vi "Curtin1_Color.vi"(8 "Offset":u16, 10 "Files in":T1[](array[typedef]), 11 "Color":u32[](array[colorbox])) -> (2 "New color":u32, 3 "Color palette":u32[](array[colorbox]))   [LabVIEW 2022 SP3]
uses:
  Curtin1_Label.ctl
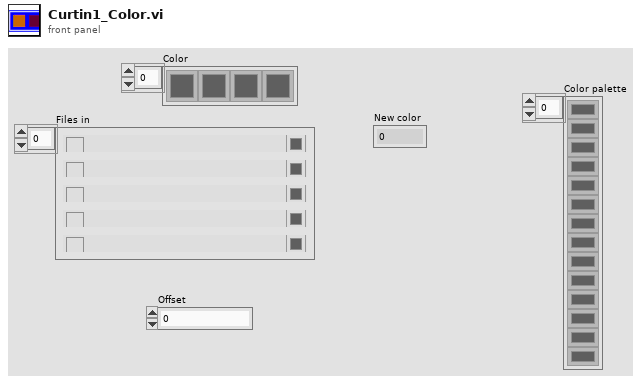
[diagram p1: front panel]
types:
  T1 = typedef "Curtin1_Label.ctl" = cluster{"Show?":bool, "Name":string, "Color":u32, "Path":path, "Show Notes":bool}
  T2 = enum16{"big-endian, network order", "native, host order", "little-endian"}
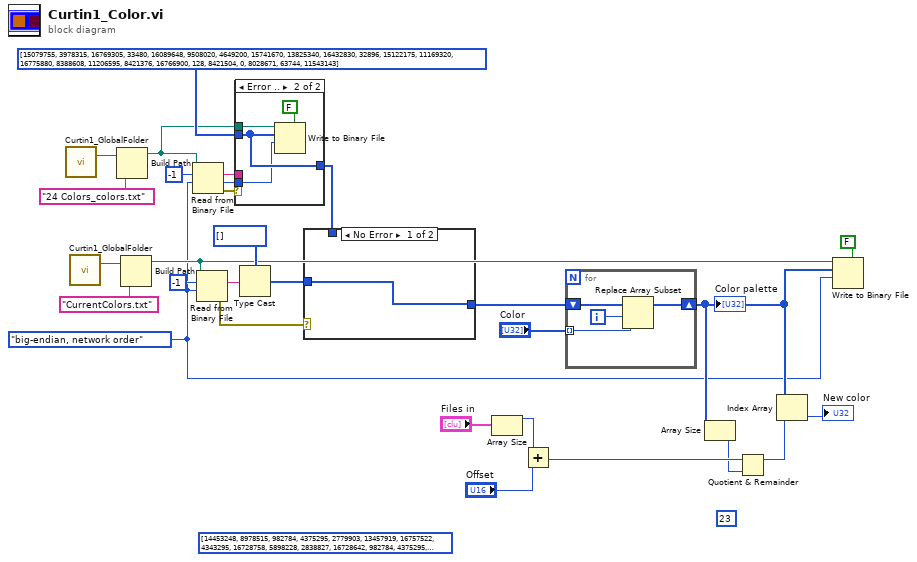
[diagram p0: block diagram]
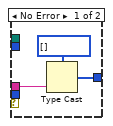
[diagram p2: hidden frame]
diagram:
  w1 = T2."big-endian, network order" ("byte order (0:big-endian, network order)")
  (unwired) 23 ("y")
  (unwired) u32[] [14453248, 8978515, 982784, 4375295, 2779903, 13457919, 16757522, 4343295, 16728758, 5898228, 2838827, 16728642, 982784, 4375295, 13827953, 13457919, 16757522, 4343295, 16728758, 5898228, 16777215, 16728642, 982784, 4375295, 13827953, 13457919, 16757522, 4343295, 16728758, 5898228, 16777215, 16728642, 982784, 4375295, 13827953, 13457919, 16757522, 4343295, 16728758, 5898228, 16777215, 16728642, 982784, 4375295, 13827953, 13457919, 16757522, 4343295, 16728758, 5898228, 16777215, 16728642, 982784, 4375295, 13827953, 13457919, 16757522, 4343295, 16728758, 5898228, 16777215, 16728642, 982784, 4375295, 13827953, 13457919, 16757522, 4343295, 16728758, 5898228, 16777215, 16728642, 982784, 4375295, 13827953, 13457919, 16757522, 4343295, 16728758, 5898228, 16777215, 16728642, 982784, 4375295, 13827953, 13457919, 16757522, 4343295, 16728758, 5898228, 16777215, 16728642, 982784, 4375295, 13827953, 13457919, 16757522, 4343295, 16728758, 5898228] ("Array")
  n1 = call "Curtin1_GlobalFolder.vi"() -> ("LabVIEW Data Path"=w9:path)  [unwired: 1 in, 1 out]
  n2 = call "Curtin1_GlobalFolder.vi"() -> ("LabVIEW Data Path"=w22:path)  [unwired: 1 in, 1 out]
  n3 = Build Path(base path=w9, name or relative path="24 Colors_colors.txt") -> (appended path=w2:path)
  n4 = Build Path(base path=w22, name or relative path="CurrentColors.txt") -> (appended path=w15:path)
  n5 = Read from Binary File(9:w1, 10:-1 ("count (1)"), 11:w2) -> (0:w5:errorcluster, 2:w11:string)  [unwired: 3 in, 2 out]
  n6 = Read from Binary File(9:w1, 10:-1 ("count (1)"), 11:w15) -> (0:w20:errorcluster, 2:w18:string)  [unwired: 3 in, 2 out]
  n7 = case shown="Error .." w5 {
    tunnel: w11 -> [w30 _]
    tunnel: [w29 w34] -> w4
    tunnel: u32[] [15079755, 3978315, 16769305, 33480, 16089648, 9508020, 4649200, 15741670, 13825340, 16432830, 32896, 15122175, 11169320, 16775880, 8388608, 11206595, 8421376, 16766900, 128, 8421504, 0, 8028671, 63744, 11543143] ("Colors") -> [_ w34]
    tunnel: w2 -> [_ w33]
    tunnel: w1 -> [_ w32]
    frame No Error {
      n8 = Type Cast(type=u32[] [] ("Color"), x=w30) -> (*(type *) &x=w29:u32[])
    }
    frame Error {
      n9 = Write to Binary File(file (use dialog)=w33, data=w34, 5:FALSE ("prepend array or string size? (T)"), 9:w32) -> ()  [unwired: 2 in, 3 out]
    }
  }
  n10 = Type Cast(type=u32[] [] ("Color"), x=w18) -> (*(type *) &x=w16:u32[])
  n11 = case shown="No Error" w20 {
    tunnel: [w36 w37] -> w19
    tunnel: w4 -> [_ w37]
    tunnel: w16 -> [w36 _]
    frame No Error {
    }
    frame Error {
    }
  }
  n12 = Array Size(array="Files in") -> (size(s)=w25:i32)
  n13 = Add(x=w25, y="Offset") -> (x+y=w24:i32)
  n14 = for {
    shift-right: [w40] -> w7
    shift-left: w19 -> [w41]
    tunnel: "Color" -> [w38] mode=indexing
    i -> [w39]
    n15 = Replace Array Subset(array=w41, new element=w38, index=w39) -> (w40:u32[])
  }
  "Color palette" <- w7
  n16 = Array Size(array=w7) -> (size(s)=w6:i32)
  n17 = Quotient & Remainder(x=w24, y=w6) -> (x-y*floor(x/y)=w14:i32)  [unwired: 1 out]
  n18 = Index Array(array=w7, index=w14) -> (element=→"New color":u32)
  n19 = Write to Binary File(file (use dialog)=w15, data=w7, 5:FALSE ("prepend array or string size? (T)"), 9:w1) -> ()  [unwired: 2 in, 3 out]
